vi "Open.vi"(0 "config":T3, 11 "error in (no error)":errorcluster) -> (4 "reference":T1, 15 "error out":errorcluster)   [LabVIEW 2017, in "JSON_RPC_client.lvlib"]
uses:
  JSON_RPC_client.lvlib
  config.ctl
  reference.ctl
  <vilib>/httpClient/ClientHandle.ctl
  <vilib>/httpClient/LabVIEWHTTPClient.lvlib
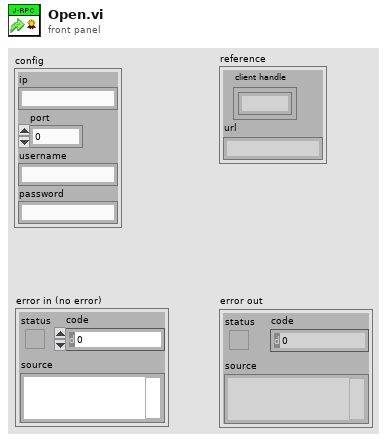
[diagram p1: front panel]
types:
  T1 = typedef "JSON_RPC_client.lvlib/reference.ctl" = cluster{"client handle":T2, "url":string}
  T2 = typedef "LabVIEWHTTPClient.lvlib/ClientHandle.ctl" = refnum<k1>
  T3 = typedef "JSON_RPC_client.lvlib/config.ctl" = cluster{"ip":string, "port":i32, "username":string, "password":string}
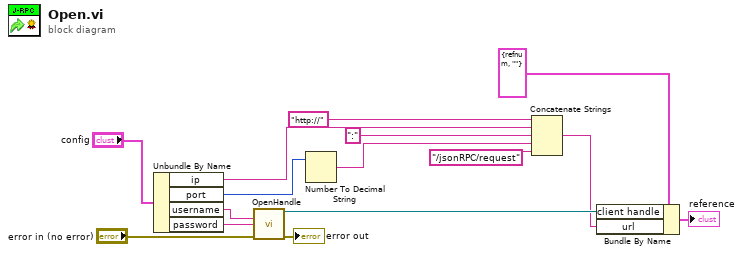
[diagram p0: block diagram]
diagram:
  n1 = Unbundle By Name("config") -> ("ip"=w10:string, "port"=w8:i32, "username"=w13:string, "password"=w12:string)
  n2 = call <vilib>:"OpenHandle.vi"("username"=w13, "password"=w12, "error in (no error)"="error in (no error)") -> ("client handle out"=w4:T2, "error out"=→"error out":errorcluster)  [unwired: 11 in]
  n3 = Number To Decimal String(number=w8) -> (decimal integer string=w7:string)  [unwired: 1 in]
  n4 = Concatenate Strings("http://", w10, ":" ("string"), w7, "/jsonRPC/request" ("string")) -> (w3:string)
  n5 = Bundle By Name(cluster=T1 {"client handle"=refnum, "url"=""} ("reference"), "client handle"=w4, "url"=w3) -> (→"reference":T1)
